vi "USBImageContinuousV1.1.vi"() -> ()   [LabVIEW 2017]
uses:
  <vilib>/Utility/file.llb/Write Delimited Spreadsheet (I64).vi
  atmcd32d.dll
panel:
  in  "Tab Control":T1(tab)
  out "Expected position on spectrometer (pixels):":dbl
  in  "Harmonic":dbl min=10.0 max=40.0
  out "l (nm)":dbl
  out "E (J)":dbl
  out "E (eV)":dbl
  out "Nearest Harmonic of 800nm":dbl
  out "Cursor Position (pixels)":dbl
  out "Distance to nearest harmonic of 800nm (pixels)":dbl
  in  "Grating:":u16(ring) items=["Shimadzu 30-006  "]
  in  "Laser:":u16(ring) items=["800nm  "]
  in  "Trigger":u32(ring) items=["Internal", "External"]
  out "Initialize":u32
  in  "Exposure Time (secs)":sgl format="%.2f"
  out "Calculated Exposure Value":sgl format="%.5f"
  out "Get Acquired Data":u32
  out "Start Acquisition":u32
  out "Detector X Pixels":i32
  out "Check Timings":u32
  out "Set Acquisition Mode":u32
  out "Set Readout Mode":u32
  out "Set Trigger Mode":u32
  out "Set Exposure Time":u32
  out "Get Detector":u32
  out "Detector Y Pixels":i32
  out "Shut Down":u32
  out "Set Gate Mode":u32
  out "Set Image":u32
  out "Intensity Graph":i32[][](graph)
  out "Vertical Binned Waveform Graph":i32[](graph)
  out "Get Status":u32
  in  "Stop":bool
  in  "?":bool
  out "Camera Status:":bool
  out "Last Image Saved:":string
  out "Wavelength Graph":cluster{"No prefix":dbl, i32}[](graph)
  out "Energy Graph (eV)":cluster{"eV":dbl, i32}[](graph)
  out "Harmonics Graph":cluster{"No prefix":dbl, i32}[](graph)
  out "Status":u32
  # "Status"
  # "Return values"
  # "USB iStarIMAG32at.VI"
  # "Acquisition Mode: Single Scan\nReadout Mode: Full Resolution Image"
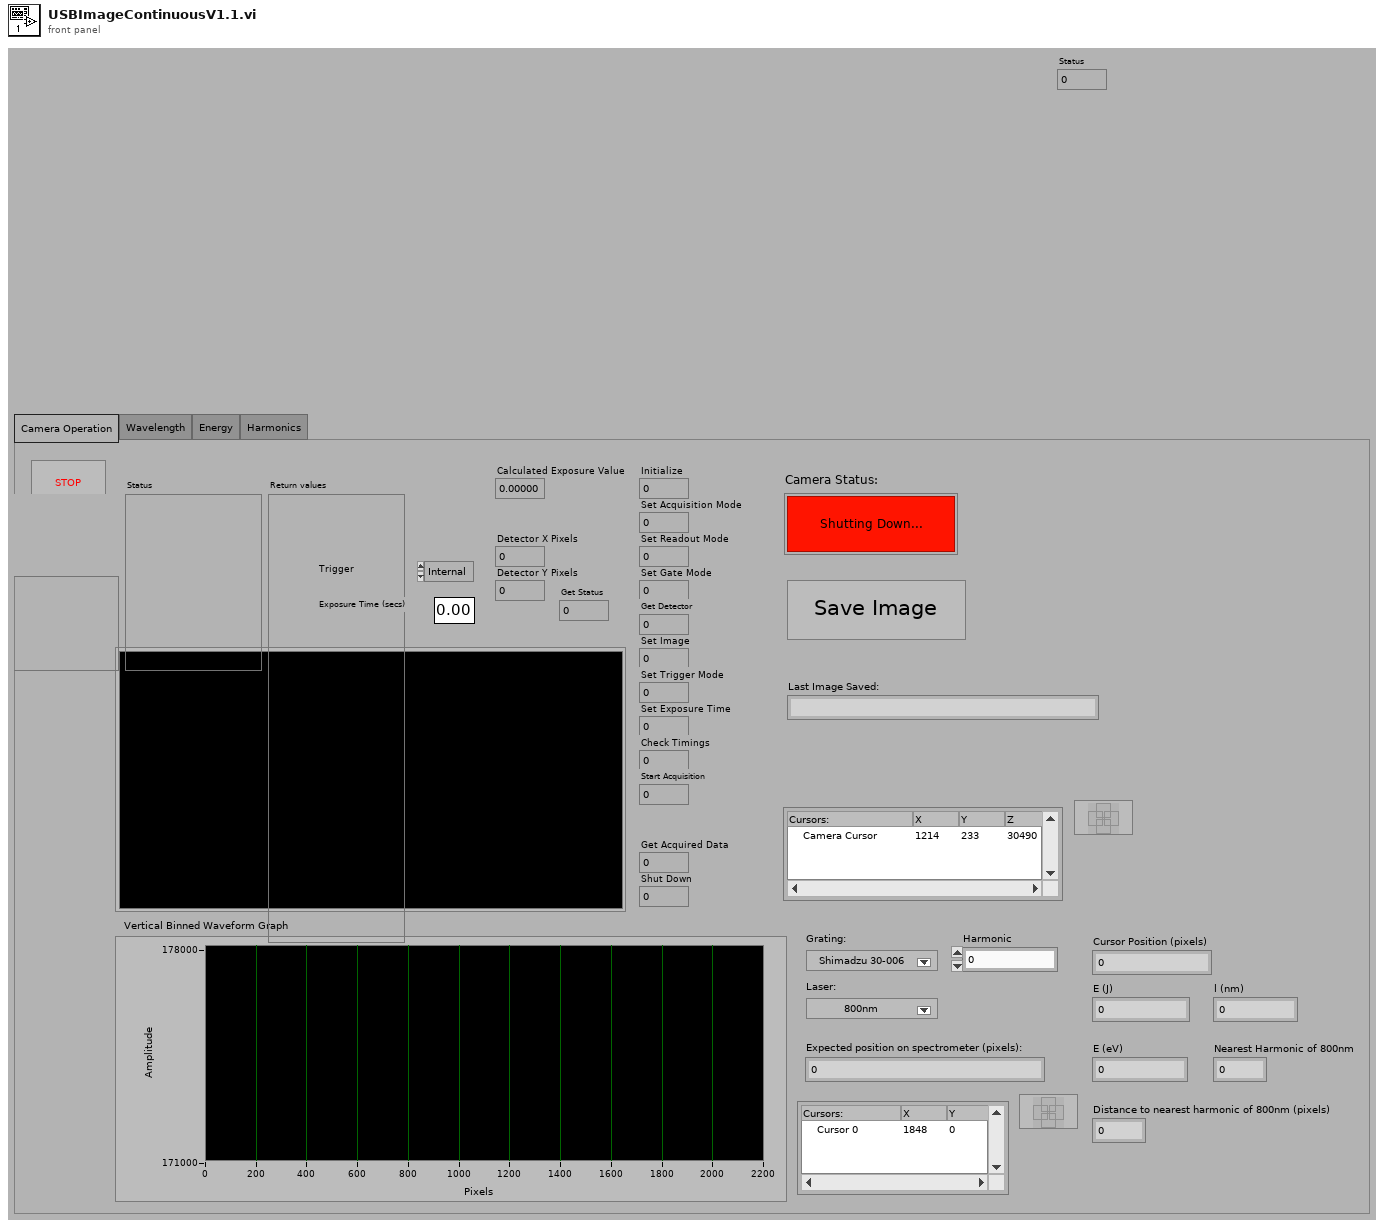
[diagram p1: front panel]
types:
  T1 = enum32{"Camera Operation", "Wavelength", "Energy", "Harmonics"}
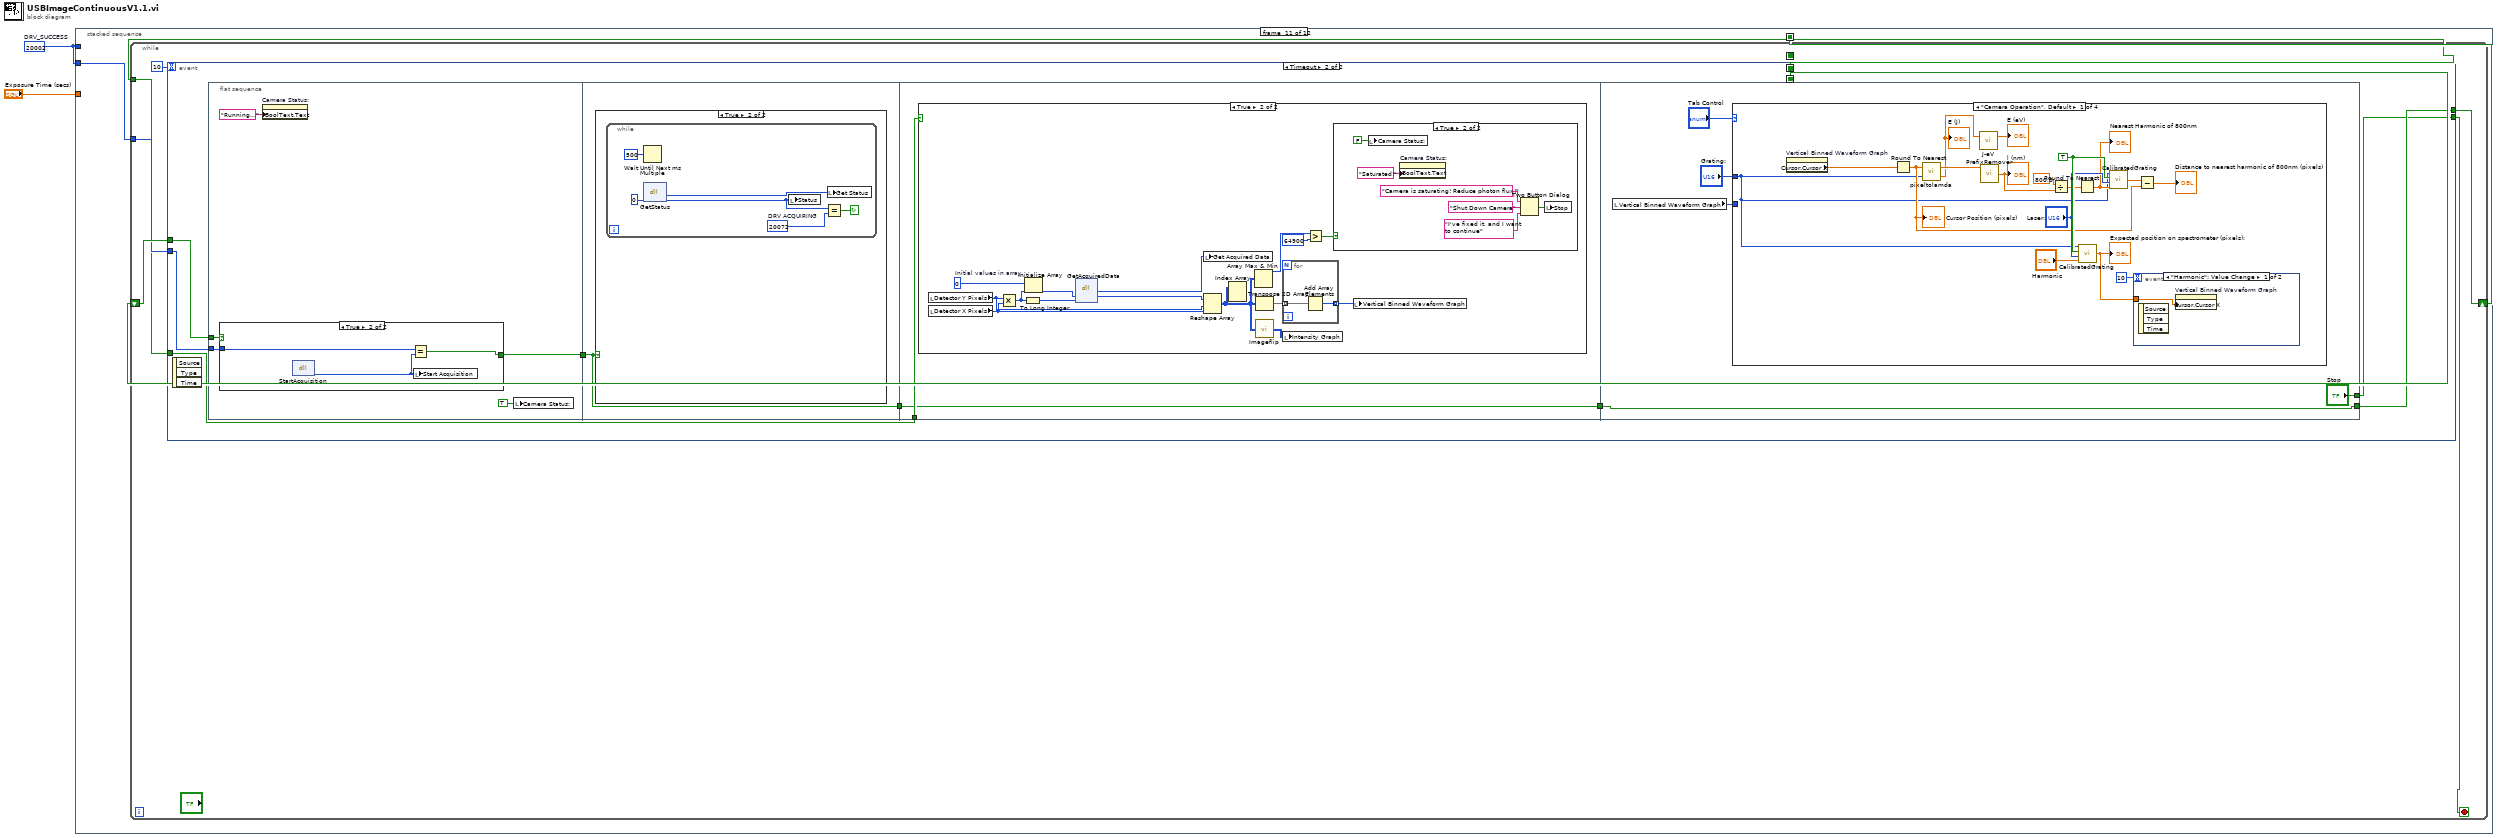
[diagram p0: block diagram]
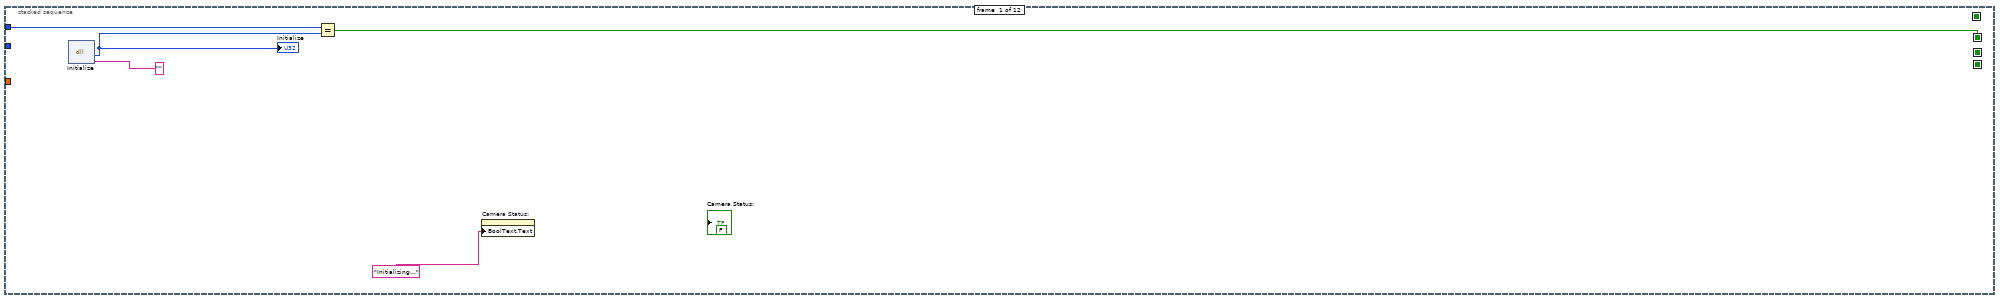
[diagram p2: hidden frame]
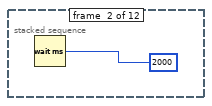
[diagram p3: hidden frame]
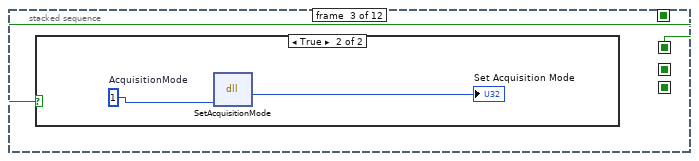
[diagram p4: hidden frame]
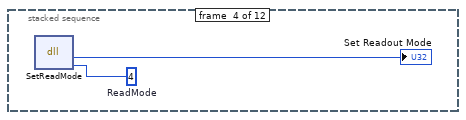
[diagram p6: hidden frame]
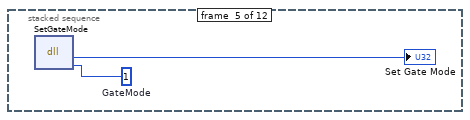
[diagram p7: hidden frame]
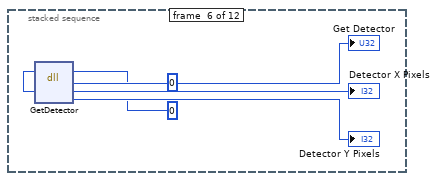
[diagram p8: hidden frame]
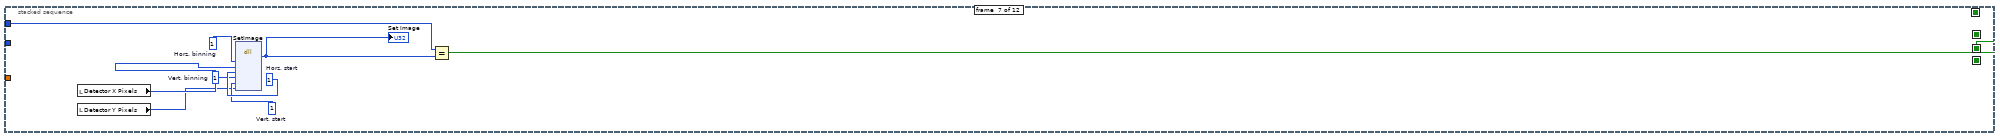
[diagram p9: hidden frame]
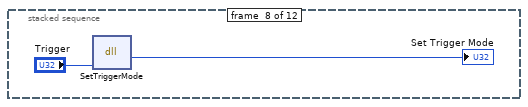
[diagram p10: hidden frame]
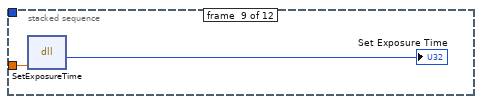
[diagram p11: hidden frame]
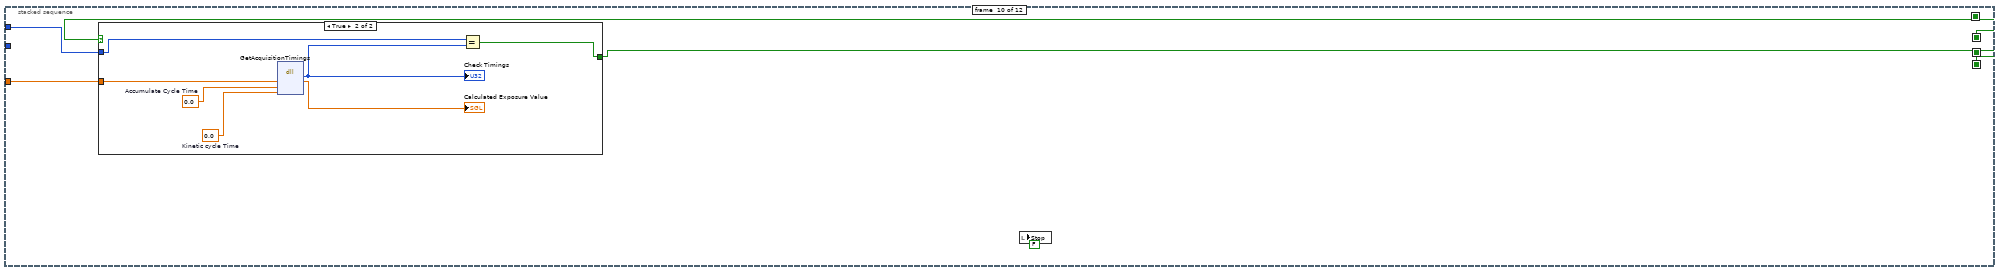
[diagram p12: hidden frame]
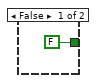
[diagram p13: hidden frame]
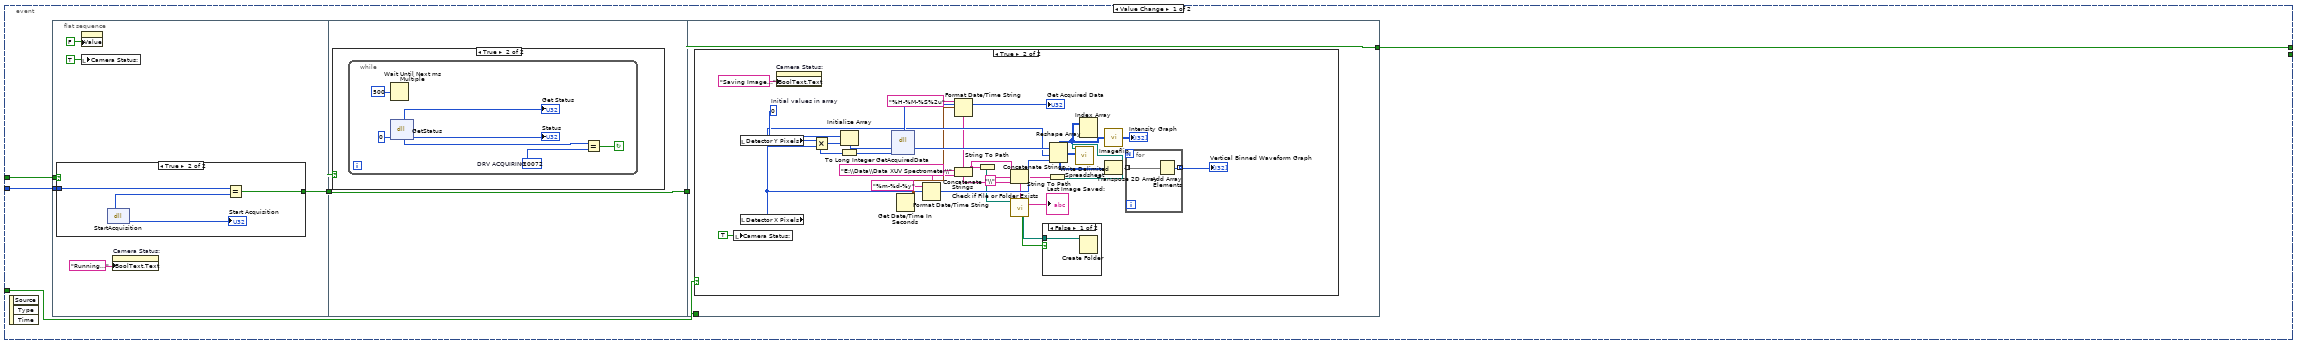
[diagram p14: hidden frame]
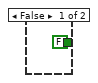
[diagram p15: hidden frame]
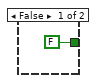
[diagram p19: hidden frame]
diagram:
  w1 = 20002  # DRV_SUCCESS
  n1 = stacked-sequence {
    seq-local: [w6 _ _ _ _ _ _ _ _ _ _ _] -> [_ _ w10 _ _ _ _ _ _ w36 _ w218]
    seq-local: [_ _ _ _ _ _ _ _ _ w37 _ _] -> [_ _ _ _ _ _ _ _ _ _ w51 _]
    seq-local: [_ _ _ _ _ _ _ _ _ _ w49 _] -> [_ _ _ _ _ _ _ _ _ _ _ _]
    seq-local: [_ _ _ _ _ _ w22 _ _ _ _ _] -> [_ _ _ _ _ _ _ _ _ _ w48 _]
    tunnel: "Exposure Time (secs)" -> [_ _ _ _ _ _ _ _ w34 w39 _ _]
    tunnel: w1 -> [w7 _ _ _ _ _ w24 _ _ w38 _ _]
    tunnel: w1 -> [_ _ _ _ _ _ _ _ _ _ w50 _]
    frame #0 {
      n2 = dll-call lib="atmcd32d.dll" fn="Initialize" label="Call Library Function Initialize"("") -> (w8:u32)  [unwired: 4 in, 2 out]
      "Initialize" <- w8
      n3 = Equal?(x=w7, y=w8) -> (x = y?=w6:bool)
      n4 = property on="Camera Status:" class="Bool (strict)"("BoolText.Text"="Initializing..." ("String")) -> ()  [unwired: 2 in, 2 out]
      "Camera Status:" <- FALSE ("Camera Status:")
    }
    frame #1 {
      n5 = Wait (ms)(milliseconds to wait=u32 2000) -> ()  [unwired: 1 out]
    }
    frame #2 {
      n6 = case shown="True" w10 {
        frame False {
        }
        frame True {
          w12 = u16 1  # AcquisitionMode
          n7 = dll-call lib="atmcd32d.dll" fn="SetAcquisitionMode" label="Call Library Function SetAcquisitionMode"(w12) -> (→"Set Acquisition Mode":u32)  [unwired: 4 in, 2 out]
        }
      }
    }
    frame #3 {
      w14 = u16 4  # ReadMode
      n8 = dll-call lib="atmcd32d.dll" fn="SetReadMode" label="Call Library Function SetReadMode"(w14) -> (→"Set Readout Mode":u32)  [unwired: 4 in, 2 out]
    }
    frame #4 {
      w16 = u16 1  # GateMode
      n9 = dll-call lib="atmcd32d.dll" fn="SetGateMode" label="Call Library Function SetGateMode"(w16) -> (→"Set Gate Mode":u32)  [unwired: 4 in, 2 out]
    }
    frame #5 {
      n10 = dll-call lib="atmcd32d.dll" fn="GetDetector" label="Call Library FunctionGetDetector"(i16 0, i16 0) -> (→"Get Detector":u32, →"Detector X Pixels":i32, →"Detector Y Pixels":i32)  [unwired: 3 in, 2 out]
    }
    frame #6 {
      w27 = u16 1  # Vert. start
      w28 = u16 1  # Horz. start
      w29 = u16 1  # Vert. binning
      w30 = u16 1  # Horz. binning
      n11 = local read "Detector X Pixels"() -> (w26:i32)
      n12 = local read "Detector Y Pixels"() -> (w25:i32)
      n13 = dll-call lib="atmcd32d.dll" fn="SetImage" label="Call Library Function SetImage"(w30, w29, w28, w26, w27, w25) -> (w23:u32)  [unwired: 9 in, 2 out]
      "Set Image" <- w23
      n14 = Equal?(x=w24, y=w23) -> (x = y?=w22:bool)
    }
    frame #7 {
      n15 = dll-call lib="atmcd32d.dll" fn="SetTriggerMode" label="Call Library Function SetTrigger Mode"("Trigger") -> (→"Set Trigger Mode":u32)  [unwired: 4 in, 2 out]
    }
    frame #8 {
      n16 = dll-call lib="atmcd32d.dll" fn="SetExposureTime" label="Call Library FunctionSet Exposure Time"(w34) -> (→"Set Exposure Time":u32)  [unwired: 4 in, 2 out]
    }
    frame #9 {
      n17 = case shown="True" w36 {
        tunnel: w39 -> [_ w44]
        tunnel: w38 -> [_ w41]
        tunnel: [FALSE w43] -> w37
        frame False {
        }
        frame True {
          w46 = sgl 0.0  # Accumulate Cycle Time
          w47 = sgl 0.0  # Kinetic cycle Time
          n18 = dll-call lib="atmcd32d.dll" fn="GetAcquisitionTimings" label="Call Library Function Check Timings"(w44, w46, w47) -> (w42:u32, →"Calculated Exposure Value":sgl)  [unwired: 5 in, 2 out]
          "Check Timings" <- w42
          n19 = Equal?(x=w41, y=w42) -> (x = y?=w43:bool)
        }
      }
      n20 = local write "Stop"(FALSE ("Stop")) -> ()
    }
    frame #10 {
      n21 = while {
        tunnel: w50 -> [w56]
        tunnel: w48 -> [w54]
        shift-right: [w55] -> w49
        shift-left: w51 -> [w57]
        stop <- w52 stop-if-true
        n22 = event shown="[1] Timeout" {
          selector: _ -> [_ _]
          dyn-events: _ -> [_ _]
          timeout: 10 -> [_ _]
          tunnel: w57 -> [w61 w118]
          tunnel: w56 -> [w60 w117]
          tunnel: [w59 w116] -> w55
          tunnel: w54 -> [w58 w115]
          tunnel: [_ w114] -> w52
          event Value Change {
            n23 = event-data() -> ()  [unwired: 1 in, 3 out]
            n24 = flat-sequence {
              tunnel: w61 -> [w69]
              tunnel: w60 -> [w68]
              tunnel: [w67] -> w63
              tunnel: w63 -> [w74]
              tunnel: [w74] -> w62
              tunnel: [w82] -> w59
              tunnel: w62 -> [w82]
              tunnel: w58 -> [w81]
              frame #0 {
                n25 = case shown="True" w69 {
                  tunnel: [FALSE w72] -> w67
                  tunnel: w68 -> [_ w71]
                  frame False {
                  }
                  frame True {
                    n26 = dll-call lib="atmcd32d.dll" fn="StartAcquisition" label="Call Library Function start acquisition"() -> (w73:u32)  [unwired: 3 in, 2 out]
                    "Start Acquisition" <- w73
                    n27 = Equal?(x=w71, y=w73) -> (x = y?=w72:bool)
                  }
                }
                n28 = property class="Bool (strict)"("Value"=FALSE ("Take image")) -> ()  [unwired: 2 in, 2 out]
                n29 = local write "Camera Status:"(TRUE ("Camera Status:")) -> ()
                n30 = property on="Camera Status:" class="Bool (strict)"("BoolText.Text"="Running..." ("Boolean Text.Text")) -> ()  [unwired: 2 in, 2 out]
              }
              frame #1 {
                n31 = case shown="True" w74 {
                  frame False {
                  }
                  frame True {
                    n32 = while {
                      stop <- w78 continue-if-true
                      w77 = u16 20072  # DRV ACQUIRING
                      n33 = Wait Until Next ms Multiple(millisecond multiple=u32 500) -> ()  [unwired: 1 out]
                      n34 = dll-call lib="atmcd32d.dll" fn="GetStatus" label="Call Library Function GetAcquisitionStatus"(u16 0) -> (→"Get Status":u32, w76:u32)  [unwired: 3 in, 2 out]
                      "Status" <- w76
                      n35 = Equal?(x=w76, y=w77) -> (x = y?=w78:bool)
                    }
                  }
                }
              }
              frame #2 {
                n36 = case shown="True" w81 {
                  frame False {
                  }
                  frame True {
                    w109 = 0  # Initial values in array
                    n37 = local write "Camera Status:"(TRUE ("Camera Status:")) -> ()
                    n38 = local read "Detector Y Pixels"() -> (w103:i32)
                    n39 = local read "Detector X Pixels"() -> (w102:i32)
                    n40 = property on="Camera Status:" class="Bool (strict)"("BoolText.Text"="Saving Image..." ("Boolean Text.Text")) -> ()  [unwired: 2 in, 2 out]
                    n41 = Multiply(x=w103, y=w102) -> (x*y=w105:i32)
                    n42 = To Long Integer(number=w105) -> (32bit integer=w106:i32)
                    n43 = Initialize Array "Initialize Array"(w109, w105) -> (w107:i32[])
                    n44 = dll-call lib="atmcd32d.dll" fn="GetAcquiredData" label="Call Library Function Get Acquired data"(w107, w106) -> (→"Get Acquired Data":u32, w104:i32[])  [unwired: 4 in, 2 out]
                    n45 = Get Date/Time In Seconds() -> (seconds since 1Jan1904=w99:timestamp)
                    n46 = Format Date/Time String(time format string (%c)="%m-%d-%y", seconds (now)=w99) -> (date/time string=w97:string)  [unwired: 1 in]
                    n47 = Format Date/Time String(time format string (%c)="%H-%M-%S%2u", seconds (now)=w99) -> (date/time string=w98:string)  [unwired: 1 in]
                    n48 = Concatenate Strings("E:\\Data\\Data XUV Spectrometer\\" ("string"), w97) -> (w100:string)
                    n49 = String To Path(string=w100) -> (path=w96:path)
                    n50 = Concatenate Strings(w100, "\\" ("string"), w98) -> (w101:string)
                    "Last Image Saved:" <- w101
                    n51 = call <vilib>:"Check if File or Folder Exists.vi"("path"=w96) -> ("file or folder exists?"=w94:bool, "dup path"=w95:path)  [unwired: 8 in, 1 out]
                    n52 = case shown="False" w94 {
                      tunnel: w95 -> [w112 _]
                      frame False {
                        n53 = Create Folder(path (use dialog)=w112) -> ()  [unwired: 2 in, 3 out]
                      }
                      frame True {
                      }
                    }
                    n54 = String To Path(string=w101) -> (path=w89:path)
                    n55 = Reshape Array(w104, w103, w102) -> (w84:i32[][])
                    n56 = call-poly <vilib>:"Write Delimited Spreadsheet.vi"("file path (dialog if empty)"=w89, "2D data"=w84) -> ()  [unwired: 12 in, 2 out]
                    n57 = Index Array(array=w84) -> ()  [unwired: 2 in, 1 out]
                    n58 = call "Imageflip.vi"("2D array"=w84) -> ("transposed array"=→"Intensity Graph":i32[][])
                    n59 = Transpose 2D Array(2D array=w84) -> (transposed array=w88:i32[][])
                    n60 = for {
                      tunnel: w88 -> [w111] mode=indexing
                      tunnel: [w110] -> w87 mode=indexing
                      n61 = Add Array Elements(numeric array=w111) -> (sum=w110:i32)
                    }
                    "Vertical Binned Waveform Graph" <- w87
                  }
                }
              }
            }
          }
          event Timeout {
            n62 = event-data() -> ()  [unwired: 1 in, 3 out]
            n63 = flat-sequence {
              tunnel: w118 -> [w125]
              tunnel: w117 -> [w124]
              tunnel: [w123] -> w120
              tunnel: w120 -> [w130]
              tunnel: [w130] -> w119
              tunnel: w119 -> [w137]
              tunnel: w115 -> [w138]
              tunnel: [w137] -> w113
              tunnel: ["Stop"] -> w114
              tunnel: [w166] -> w116
              tunnel: w113 -> [w166]
              frame #0 {
                n64 = case shown="True" w125 {
                  tunnel: [FALSE w129] -> w123
                  tunnel: w124 -> [_ w128]
                  frame False {
                  }
                  frame True {
                    n65 = dll-call lib="atmcd32d.dll" fn="StartAcquisition" label="Call Library Function start acquisition"() -> (w127:u32)  [unwired: 3 in, 2 out]
                    n66 = Equal?(x=w128, y=w127) -> (x = y?=w129:bool)
                    n67 = local write "Start Acquisition"(w127) -> ()
                  }
                }
                n68 = property on="Camera Status:" class="Bool (strict)"("BoolText.Text"="Running..." ("Boolean Text.Text")) -> ()  [unwired: 2 in, 2 out]
                n69 = local write "Camera Status:"(TRUE ("Camera Status:")) -> ()
              }
              frame #1 {
                n70 = case shown="True" w130 {
                  frame False {
                  }
                  frame True {
                    n71 = while {
                      stop <- w134 continue-if-true
                      w133 = u16 20072  # DRV ACQUIRING
                      n72 = Wait Until Next ms Multiple(millisecond multiple=u32 500) -> ()  [unwired: 1 out]
                      n73 = dll-call lib="atmcd32d.dll" fn="GetStatus" label="Call Library Function GetAcquisitionStatus"(u16 0) -> (w132:u32, w131:u32)  [unwired: 3 in, 2 out]
                      n74 = local write "Status"(w131) -> ()
                      n75 = Equal?(x=w131, y=w133) -> (x = y?=w134:bool)
                      n76 = local write "Get Status"(w132) -> ()
                    }
                  }
                }
              }
              frame #2 {
                n77 = case shown="True" w138 {
                  frame False {
                  }
                  frame True {
                    w153 = 0  # Initial values in array
                    n78 = local read "Detector Y Pixels"() -> (w148:i32)
                    n79 = local read "Detector X Pixels"() -> (w147:i32)
                    n80 = Multiply(x=w148, y=w147) -> (x*y=w150:i32)
                    n81 = To Long Integer(number=w150) -> (32bit integer=w151:i32)
                    n82 = Initialize Array "Initialize Array"(w153, w150) -> (w152:i32[])
                    n83 = dll-call lib="atmcd32d.dll" fn="GetAcquiredData" label="Call Library Function Get Acquired data"(w152, w151) -> (w145:u32, w149:i32[])  [unwired: 4 in, 2 out]
                    n84 = local write "Get Acquired Data"(w145) -> ()
                    n85 = Reshape Array(w149, w148, w147) -> (w139:i32[][])
                    n86 = Index Array(array=w139) -> ()  [unwired: 2 in, 1 out]
                    n87 = Array Max & Min(array=w139) -> (max value=w143:i32)  [unwired: 3 out]
                    n88 = Transpose 2D Array(2D array=w139) -> (transposed array=w146:i32[][])
                    n89 = call "Imageflip.vi"("2D array"=w139) -> ("transposed array"=w140:i32[][])
                    n90 = for {
                      tunnel: w146 -> [w161] mode=indexing
                      tunnel: [w160] -> w144 mode=indexing
                      n91 = Add Array Elements(numeric array=w161) -> (sum=w160:i32)
                    }
                    n92 = local write "Intensity Graph"(w140) -> ()
                    n93 = Greater?(x=w143, y=64900) -> (0:w141:bool)
                    n94 = case shown="True" w141 {
                      frame False {
                      }
                      frame True {
                        n95 = local write "Camera Status:"(FALSE ("Camera Status:")) -> ()
                        n96 = property on="Camera Status:" class="Bool (strict)"("BoolText.Text"="Saturated!" ("Boolean Text.Text")) -> ()  [unwired: 2 in, 2 out]
                        n97 = Two Button Dialog(message="Camera is saturating! Reduce photon flux!", 1:"I've fixed it, and I want to continue" ("message"), 2:"Shut Down Camera" ("T button name (\"OK\")")) -> (T button?=w155:bool)
                        n98 = local write "Stop"(w155) -> ()
                      }
                    }
                    n99 = local write "Vertical Binned Waveform Graph"(w144) -> ()
                  }
                }
              }
              frame #3 {
                n100 = local read "Vertical Binned Waveform Graph"() -> (w163:i32[])
                n101 = case shown="\"Camera Operation\", Default" "Tab Control" {
                  tunnel: w163 -> [_ w187 w196 w205]
                  tunnel: "Grating:" -> [w167 w186 w195 w204]
                  frame "Camera Operation", Default {
                    w183 = TRUE
                    n102 = property on="Vertical Binned Waveform Graph" class="WFGraph (strict)"() -> ("Cursor.Cursor X"=w180:dbl)  [unwired: 2 in, 2 out]
                    n103 = Round To Nearest(number=w180) -> (nearest integer value=w173:dbl)
                    "Cursor Position (pixels)" <- w173
                    n104 = call "pixeltolamda.vi"("Grating:"=w167, "Pixel Postion"=w173) -> ("E (J)"=w175:dbl, "lamda (m)"=w181:dbl)
                    "E (J)" <- w175
                    n105 = call "J-eV.vi"("J"=w175) -> ("eV"=→"E (eV)":dbl)  [unwired: 1 in, 1 out]
                    n106 = call "PrefixRemover.vi"("Nano"=w181) -> ("No prefix"=w176:dbl)  [unwired: 3 in]
                    "l (nm)" <- w176
                    n107 = Divide(x=800.0, y=w176) -> (x/y=w178:dbl)
                    n108 = Round To Nearest(number=w178) -> (nearest integer value=w172:dbl)
                    "Nearest Harmonic of 800nm" <- w172
                    n109 = call "CalibratedGrating.vi"("Harmonic"="Harmonic", "Laser:"="Laser:", "Subvi?"=w183, "Grating:"=w167) -> ("Position on spectrometer (pixels):"=w169:dbl)
                    "Expected position on spectrometer (pixels):" <- w169
                    n110 = call "CalibratedGrating.vi"("Harmonic"=w172, "Laser:"="Laser:", "Subvi?"=w183, "Grating:"=w167) -> ("Position on spectrometer (pixels):"=w171:dbl)
                    n111 = event shown="[0] \"Harmonic\": Value Change" {
                      selector: _ -> [_ _]
                      dyn-events: _ -> [_ _]
                      timeout: 10 -> [_ _]
                      tunnel: w169 -> [w184 _]
                      event "Harmonic": Value Change {
                        n112 = event-data() -> ()  [unwired: 1 in, 3 out]
                        n113 = property on="Vertical Binned Waveform Graph" class="WFGraph (strict)"("Cursor.Cursor X"=w184) -> ()  [unwired: 2 in, 2 out]
                      }
                      event Timeout {
                        n114 = event-data() -> ()  [unwired: 1 in, 3 out]
                      }
                    }
                    n115 = Subtract(x=w171, y=w173) -> (x-y=→"Distance to nearest harmonic of 800nm (pixels)":dbl)
                  }
                  frame "Wavelength" {
                    n116 = for {
                      tunnel: w187 -> [w189] mode=indexing
                      tunnel: w186 -> [w191]
                      tunnel: [w188] -> w185 mode=indexing
                      i -> [w190]
                      n117 = call "pixeltolamda.vi"("Grating:"=w191, "Pixel Postion"=w190) -> ("lamda (m)"=w192:dbl)  [unwired: 1 out]
                      n118 = call "PrefixRemover.vi"("Nano"=w192) -> ("No prefix"=w193:dbl)  [unwired: 3 in]
                      n119 = Bundle("No prefix"=w193, w189) -> (w188:cluster{"No prefix":dbl, i32})  [unwired: 1 in]
                    }
                    "Wavelength Graph" <- w185
                  }
                  frame "Energy" {
                    n120 = for {
                      tunnel: w196 -> [w198] mode=indexing
                      tunnel: w195 -> [w201]
                      tunnel: [w197] -> w194 mode=indexing
                      i -> [w202]
                      n121 = call "pixeltolamda.vi"("Grating:"=w201, "Pixel Postion"=w202) -> ("E (J)"=w200:dbl)  [unwired: 1 out]
                      n122 = call "J-eV.vi"("J"=w200) -> ("eV"=w199:dbl)  [unwired: 1 in, 1 out]
                      n123 = Bundle("eV"=w199, w198) -> (w197:cluster{"eV":dbl, i32})  [unwired: 1 in]
                    }
                    "Energy Graph (eV)" <- w194
                  }
                  frame "Harmonics" {
                    n124 = for {
                      tunnel: w205 -> [w212] mode=indexing
                      tunnel: w204 -> [w214]
                      tunnel: [w211] -> w203 mode=indexing
                      i -> [w213]
                      n125 = call "pixeltolamda.vi"("Grating:"=w214, "Pixel Postion"=w213) -> ("lamda (m)"=w215:dbl)  [unwired: 1 out]
                      n126 = call "PrefixRemover.vi"("Nano"=w215) -> ("No prefix"=w209:dbl)  [unwired: 3 in]
                      n127 = Divide(x=800.0, y=w209) -> (x/y=w208:dbl)
                      n128 = Bundle(w208, w212) -> (w211:cluster{dbl, i32})  [unwired: 1 in]
                    }
                    n129 = flat-sequence {
                      tunnel: w203 -> [w206]
                      frame #0 {
                        "Harmonics Graph" <- w206
                      }
                      frame #1 {
                        n130 = property on="Harmonics Graph" class="XYGraph (strict)"("XScale.Minimum"=9.0 ("X Scale.Range:Increment")) -> ()  [unwired: 2 in, 2 out]
                      }
                    }
                  }
                }
              }
            }
          }
        }
      }
    }
    frame #11 {
      n131 = local write "Camera Status:"(FALSE ("Camera Status:")) -> ()
      n132 = property on="Camera Status:" class="Bool (strict)"("BoolText.Text"="Shutting Down..." ("Boolean Text.Text")) -> ()  [unwired: 2 in, 2 out]
      n133 = case shown="True" w218 {
        frame False {
        }
        frame True {
          n134 = dll-call lib="atmcd32d.dll" fn="ShutDown" label="Call Library Function Shutdown"() -> (→"Shut Down":u32)  [unwired: 3 in, 2 out]
        }
      }
    }
  }
